vi "checkTimeout.vi"(8 "error in (no error)":errorcluster, 10 "ElectrometerController in":refnum<class "ElectrometerController.lvclass">, 11 "State in":refnum<class "ReadingBufferState.lvclass">) -> (0 "error out":errorcluster, 1 "timeout?":bool, 2 "ElectrometerController out":refnum<class "ElectrometerController.lvclass">, 3 "State out":refnum<class "ReadingBufferState.lvclass">)   [LabVIEW 2016, in "ReadingBufferState.lvclass"]
uses:
  ReadingBufferState.lvclass
  ElectrometerController/ElectrometerController.lvclass
  ts_electrometeruserevents/Typedefs/StateValue.ctl
  ElectrometerReading/ElectrometerReadingStatus.lvclass
  ts_electrometeruserevents/Typedefs/ElectrometerTypedefs.lvlib
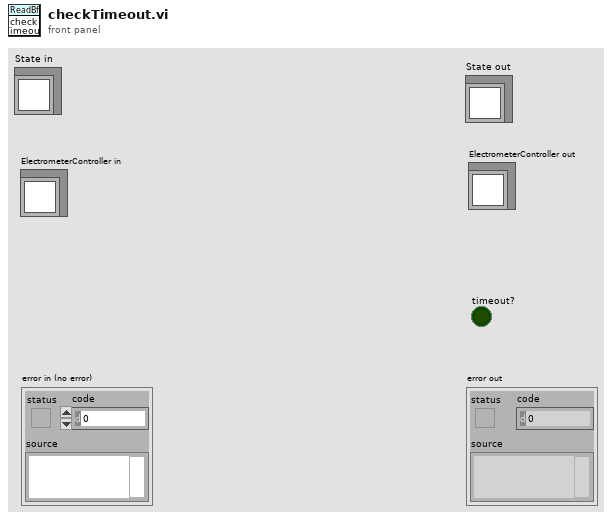
[diagram p1: front panel]
types:
  T1 = typedef "ElectrometerTypedefs.lvlib/StateValue.ctl" = enum16{"", "DisabledState", "EnabledState", "FaultState", "OffState", "StandbyState", "ReadyState", "ConfiguringState", "ManualReadingState", "UntilIntentisyReadingState", "SetDurationReadingState", "BufferReadingState"}
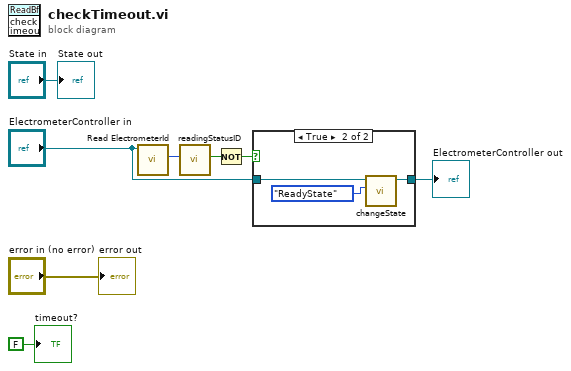
[diagram p0: block diagram]
diagram:
  n1 = call-dynamic "Read ElectrometerId.vi"("ElectrometerController in"="ElectrometerController in") -> ("ElectrometerId"=w6:enum16{"", "ID1", "ID2"})  [unwired: 8 in, 2 out]
  n2 = call "readingStatusID.vi"("ElectrometerId"=w6) -> ("Reading?"=w5:bool)  [unwired: 8 in, 2 out]
  n3 = Not(x=w5) -> (.not. x?=w1:bool)
  n4 = case shown="True" w1 {
    tunnel: [w9 w12] -> w4
    tunnel: "ElectrometerController in" -> [w9 w11]
    frame False {
    }
    frame True {
      n5 = call "changeState.vi"("StateValue"=StateValue."ReadyState", "ElectrometerController in"=w11) -> ("ElectrometerController out"=w12:refnum<class "ElectrometerController.lvclass">)  [unwired: 8 in, 1 out]
    }
  }
  "ElectrometerController out" <- w4
  "error out" <- "error in (no error)"
  "State out" <- "State in"
  "timeout?" <- FALSE ("timeout?")
